vi "createContextID.vi"(8 "error in (no error)":errorcluster, 10 "ContextID":T1, 11 "IContextIDFactory in":refnum<class "IContextIDFactory.lvclass">) -> (0 "error out":errorcluster, 2 "contextID":refnum<class "ContextID.lvclass">, 3 "IContextIDFactory out":refnum<class "IContextIDFactory.lvclass">)   [LabVIEW 2012, in "IContextIDFactory.lvclass"]
uses:
  IContextIDFactory.lvclass
  Typedefs/ContextID.ctl
  C/Program Files (x86)/National Instruments/LabVIEW 2012/user.lib/Common/ComponentModel/ComponentModel/ContextID/ContextID.lvclass
  Typedefs/EXATypedefs.lvlib
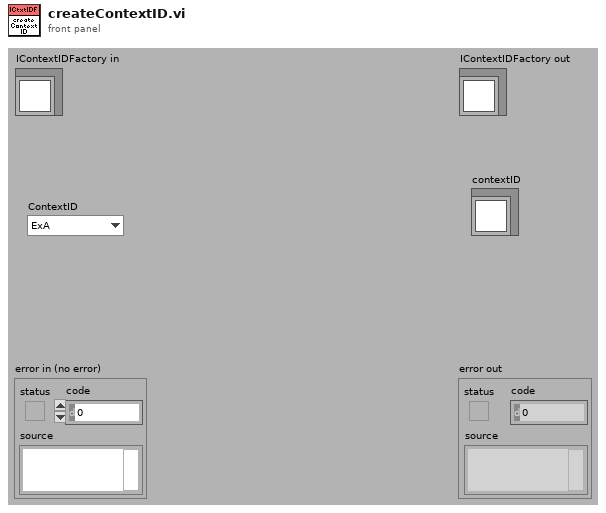
[diagram p1: front panel]
types:
  T1 = typedef "EXATypedefs.lvlib/ContextID.ctl" = enum16{"ExA"}
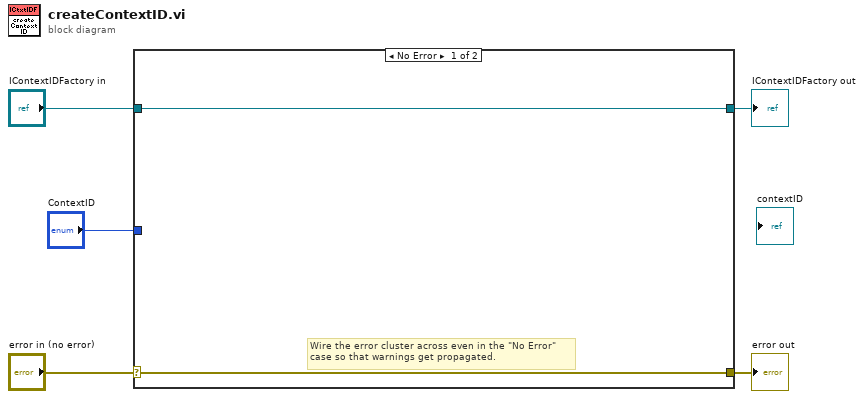
[diagram p0: block diagram]
diagram:
  n1 = case shown="No Error" "error in (no error)" {
    selector: "error in (no error)" -> [w6 w9]
    tunnel: [w6 w9] -> w4
    tunnel: [w7 w8] -> w2
    tunnel: "IContextIDFactory in" -> [w7 w8]
    tunnel: "ContextID" -> [_ _]
    frame No Error {
      # "Wire the error cluster across even in the \"No Error\"\ncase so that warnings get propagated."
    }
    frame Error {
    }
  }
  "error out" <- w4
  "IContextIDFactory out" <- w2
